vi "Decode.vi"(8 "error in (no error)":errorcluster caption="entrée d'erreur (pas d'erreur)", 9 "doc":string, 10 "X":string[][](array[string]), 11 "TfidfVectorizer.lvclass":refnum<class "TfidfVectorizer.lvclass">) -> (0 "error out":errorcluster caption="sortie d'erreur", 2 "String Data":string, 3 "TfidfVectorizer.lvclass":refnum<class "TfidfVectorizer.lvclass">)   [LabVIEW 2020, in "TfidfVectorizer.lvclass"]
doc: "Decode the input into a string of unicode symbols.\n\nThe decoding strategy depends on the vectorizer parameters.\n\nParameters : \n\n- doc : str\nThe string to decode.\n\nReturns : \n\n- doc : str\nA string of unicode symbols."
uses:
  TfidfVectorizer.lvclass
  TfidfVectorizer.lvclass/TfidfVectorizer.ctl
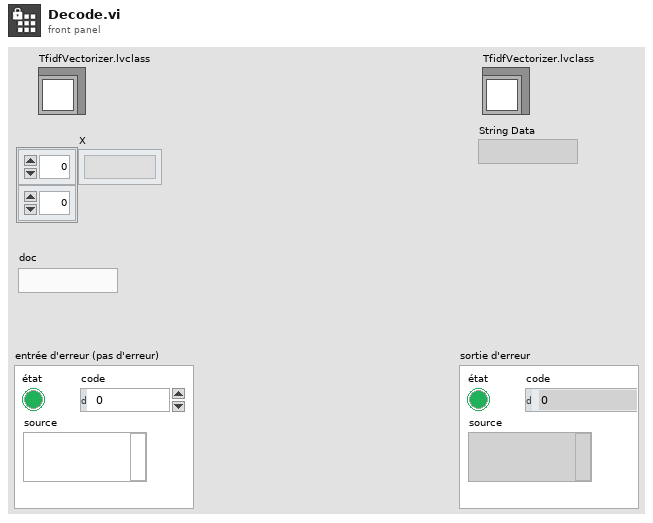
[diagram p1: front panel]
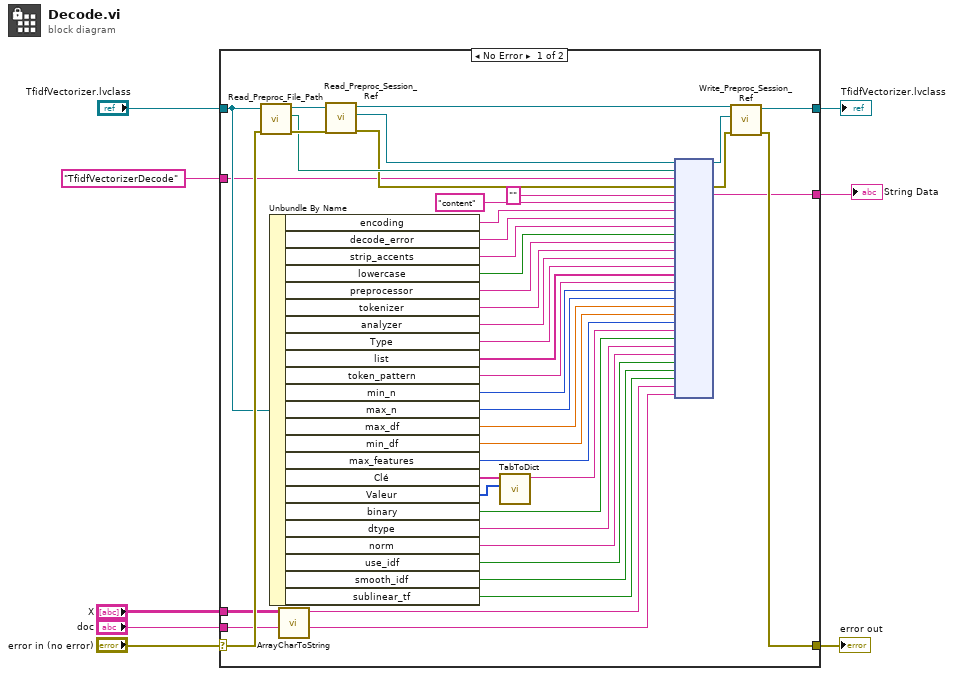
[diagram p0: block diagram]
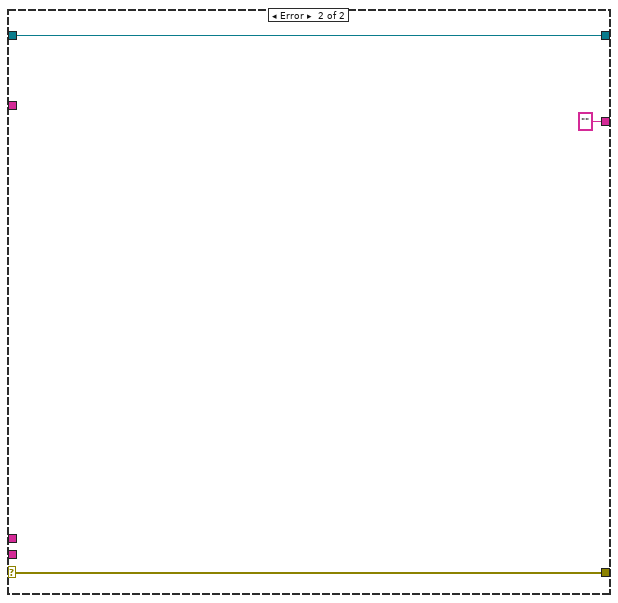
[diagram p2: hidden frame]
diagram:
  n1 = case shown="No Error" "error in (no error)" {
    selector: "error in (no error)" -> [w38 w54]
    tunnel: [w39 w54] -> w7
    tunnel: [w40 w53] -> w5
    tunnel: "TfidfVectorizer.lvclass" -> [w37 w53]
    tunnel: "TfidfVectorizerDecode" ("Fonction") -> [w36 _]
    tunnel: [w35 ""] -> w3
    tunnel: "X" -> [w10 _]
    tunnel: "doc" -> [w11 _]
    frame No Error {
      n2 = call-dynamic "Read_Preproc_File_Path.vi"("error in (no error)"=w38, "Python in"=w37) -> ("error out"=w50:errorcluster, "File_Path"=w49:path, "Python out"=w51:refnum<class "TfidfVectorizer.lvclass">)  [unwired: 7 in]
      n3 = Unbundle By Name(w37) -> ("encoding"=w42:string, "decode_error"=w41:string, "strip_accents"=w34:string, "lowercase"=w33:bool, "preprocessor"=w32:string, "tokenizer"=w31:string, "analyzer"=w30:string, "Type"=w28:string, "list"=w27:string[], "token_pattern"=w26:string, "min_n"=w25:i32, "max_n"=w24:i32, "max_df"=w23:dbl, "min_df"=w22:dbl, "max_features"=w21:i32, "Clé"=w20:string[], "Valeur"=w19:i32[], "binary"=w17:bool, "dtype"=w16:string, "norm"=w15:string, "use_idf"=w14:bool, "smooth_idf"=w13:bool, "sublinear_tf"=w12:bool)
      n4 = call "ArrayCharToString.vi"("TAB"=w10) -> ("Instruction"=w9:string)  [unwired: 10 in]
      n5 = call-dynamic "Read_Preproc_Session_Ref.vi"("error in (no error)"=w50, "Python in"=w51) -> ("error out"=w47:errorcluster, "Session_ref"=w48:refnum<k35>, "Python out"=w46:refnum<class "TfidfVectorizer.lvclass">)  [unwired: 7 in]
      n6 = call "TabToDict.vi"("Int Value"=w19, "String key"=w20) -> ("Dict with int value"=w18:string)  [unwired: 8 in, 1 out]
      n7 = node(w48, w49, w36, w47, "", "content", w42, w41, w34, w33, w32, w31, w30, w28, w27, w26, w25, w24, w23, w22, w21, w18, w17, w16, w15, w14, w13, w12, w9, w11) -> (w44:refnum<k35>, w45:errorcluster, w35:string)  [unwired: 25 in, 2 out]
      n8 = call-dynamic "Write_Preproc_Session_Ref.vi"("error in (no error)"=w45, "Session_ref"=w44, "Python in"=w46) -> ("error out"=w39:errorcluster, "Python out"=w40:refnum<class "TfidfVectorizer.lvclass">)  [unwired: 7 in]
    }
    frame Error {
    }
  }
  "error out" <- w7
  "TfidfVectorizer.lvclass" <- w5
  "String Data" <- w3
